vi "2019-05-013_EventStructure_01.vi"() -> ()   [LabVIEW 2018]
panel:
  out "숫자형 인디케이터":dbl
  in  "숫자형 컨트롤":dbl
  in  "Stop":bool
  in  "Save":bool
  in  "Open":bool
  in  "New":bool
  in  "정지":bool
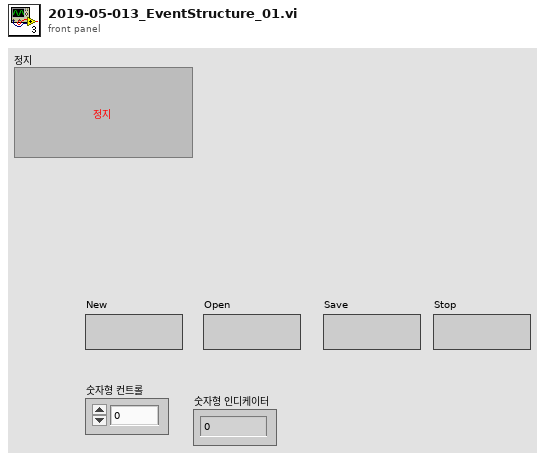
[diagram p1: front panel]
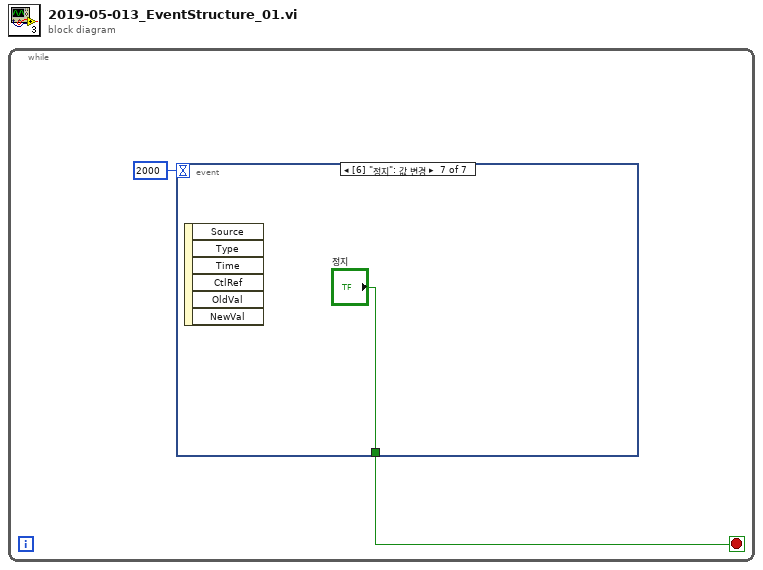
[diagram p0: block diagram]
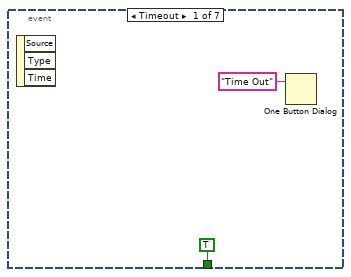
[diagram p2: hidden frame]
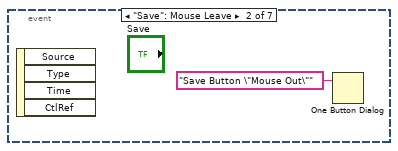
[diagram p3: hidden frame]
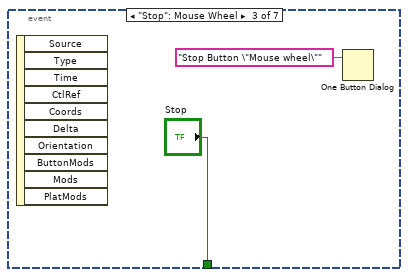
[diagram p4: hidden frame]
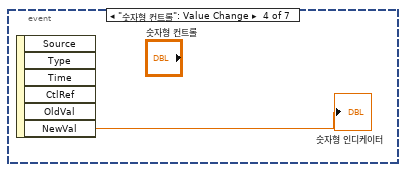
[diagram p5: hidden frame]
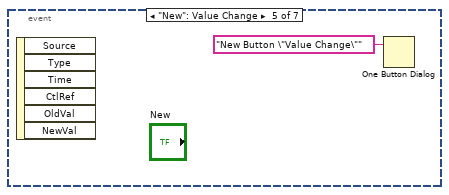
[diagram p6: hidden frame]
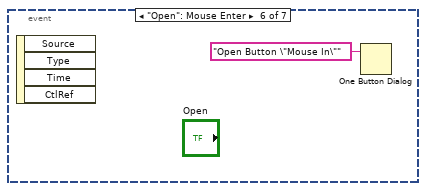
[diagram p7: hidden frame]
diagram:
  n1 = while {
    stop <- w2 stop-if-true
    n2 = event shown="[6] \"정지\": 값 변경" {
      selector: _ -> [_ _ _ _ _ _ _]
      dyn-events: _ -> [_ _ _ _ _ _ _]
      timeout: 2000 -> [_ _ _ _ _ _ _]
      tunnel: [TRUE ("정지") _ "Stop" _ _ _ "정지"] -> w2
      event Timeout {
        n3 = event-data() -> ()  [unwired: 1 in, 3 out]
        n4 = One Button Dialog(message="Time Out" ("메시지")) -> ()  [unwired: 1 in, 1 out]
      }
      event "Save": Mouse Leave {
        n5 = event-data() -> ()  [unwired: 1 in, 4 out]
        n6 = One Button Dialog(message="Save Button \"Mouse Out\"" ("메시지")) -> ()  [unwired: 1 in, 1 out]
      }
      event "Stop": Mouse Wheel {
        n7 = event-data() -> ()  [unwired: 1 in, 10 out]
        n8 = One Button Dialog(message="Stop Button \"Mouse wheel\"" ("메시지")) -> ()  [unwired: 1 in, 1 out]
      }
      event "숫자형 컨트롤": Value Change {
        n9 = event-data() -> ("NewVal"=→"숫자형 인디케이터":dbl)  [unwired: 1 in, 5 out]
      }
      event "New": Value Change {
        n10 = event-data() -> ()  [unwired: 1 in, 6 out]
        n11 = One Button Dialog(message="New Button \"Value Change\"" ("메시지")) -> ()  [unwired: 1 in, 1 out]
      }
      event "Open": Mouse Enter {
        n12 = event-data() -> ()  [unwired: 1 in, 4 out]
        n13 = One Button Dialog(message="Open Button \"Mouse In\"" ("메시지")) -> ()  [unwired: 1 in, 1 out]
      }
      event "정지": Value Change {
        n14 = event-data() -> ()  [unwired: 1 in, 6 out]
      }
    }
  }
